vi "test_Teardown_Testenvironment.vi"(8 "error in":errorcluster, 11 "horiba.lvlib:GenericDevice":refnum<class "GenericDevice.lvclass">) -> (0 "error out":errorcluster, 2 "device is open?":bool)   [LabVIEW 2023]
uses:
  Classes/DeviceManager/DeviceManager.lvlib
  Classes/GenericDevice/GenericDevice.lvclass
panel:
  # "Connector Pane"
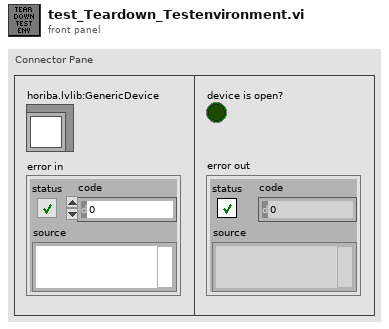
[diagram p1: front panel]
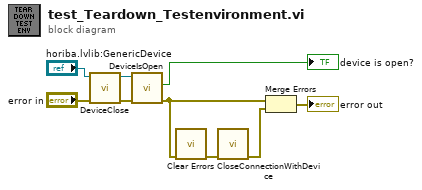
[diagram p0: block diagram]
diagram:
  n1 = call-dynamic "DeviceClose.vi"("error in (no error)"="error in", "GenericDevice in"="horiba.lvlib:GenericDevice") -> ("error out"=w7:errorcluster, "GenericDevice out"=w8:refnum<class "GenericDevice.lvclass">)  [unwired: 5 in, 3 out]
  n2 = call-dynamic "DeviceIsOpen.vi"("error in (no error)"=w7, "GenericDevice in"=w8) -> ("error out"=w3:errorcluster, "device is open?"=→"device is open?":bool)  [unwired: 6 in, 2 out]
  n3 = call <vilib>:"Clear Errors.vi"("error in (no error)"=w3) -> ("error out"=w4:errorcluster)  [unwired: 5 in, 1 out]
  n4 = call "CloseConnectionWithDevice.vi"("error in (no error)"=w4) -> ("error out"=w1:errorcluster)  [unwired: 10 in]
  n5 = Merge Errors(w3, w1) -> (→"error out":errorcluster)
